vi "Is Path to Actor.vi"(8 "error in (no error)":errorcluster, 10 "Target":refnum<vi>, 11 "Path":path) -> (0 "error out":errorcluster, 1 "Default Actor Path":path, 2 "Is Path to Actor?":bool)   [LabVIEW 2021, in "Message Maker.lvlib"]
uses:
  Message Maker.lvlib
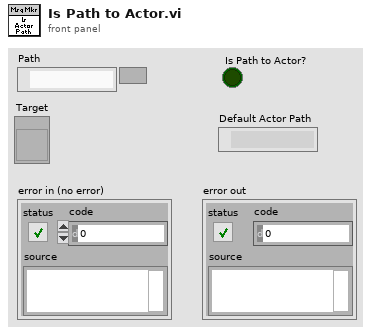
[diagram p1: front panel]
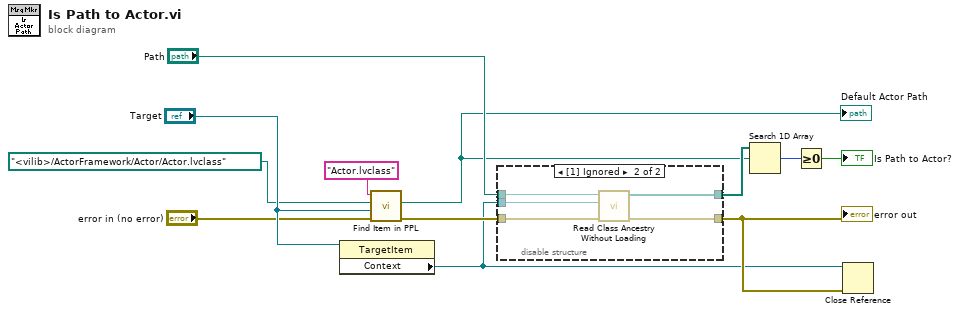
[diagram p0: block diagram]
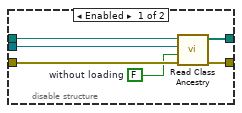
[diagram p2: hidden frame]
diagram:
  n1 = property class="TargetItem"(reference="Target") -> ("Context"=w3:refnum<vi>)  [unwired: 1 in, 2 out]
  n2 = call "Find Item in PPL.vi"("error in (no error)"="error in (no error)", "Target"="Target", "default path"=path "<vilib>/ActorFramework/Actor/Actor.lvclass", "qualified name"="Actor.lvclass") -> ("error out"=w8:errorcluster, "item path out"=w7:path)  [unwired: 5 in, 1 out]
  "Default Actor Path" <- w7
  n3 = disable-structure shown="[1] Ignored" {
    disable-tunnel: [w18 w23] -> w10
    disable-tunnel: "Path" -> [w17 w21]
    disable-tunnel: w8 -> [w16 w19]
    disable-tunnel: [w15 w22] -> w4
    disable-tunnel: w3 -> [w14 w20]
    frame Enabled {
      w13 = FALSE  # without loading
      n4 = call <vilib>:"Read Class Ancestry.vi"("error in (no error)"=w16, "without loading"=w13, "App Reference (this app)"=w14, "LabVIEW Class Path"=w17) -> ("error out"=w15:errorcluster, "Class Ancestry"=w18:path[])  [unwired: 6 in]
    }
    frame Disabled {
      n5 = call <vilib>:"Read Class Ancestry Without Loading.vi"("error in (no error)"=w19, "App Reference (this app)"=w20, "LabVIEW Class Path"=w21) -> ("error out"=w22:errorcluster, "Class Ancestry"=w23:path[])  [unwired: 7 in]
    }
  }
  "error out" <- w4
  n6 = Search 1D Array(1D array=w10, element=w7) -> (index of element=w12:i32)  [unwired: 1 in]
  n7 = Greater Or Equal To 0?(x=w12) -> (x >= 0?=→"Is Path to Actor?":bool)
  n8 = Close Reference(reference=w3, error in (no error)=w4) -> ()  [unwired: 1 out]
